vi "7-2.vi"() -> ()   [LabVIEW 2017]
panel:
  out "Gauge":dbl(knob) scale=0.0..10.0
  in  "Stop Button":bool
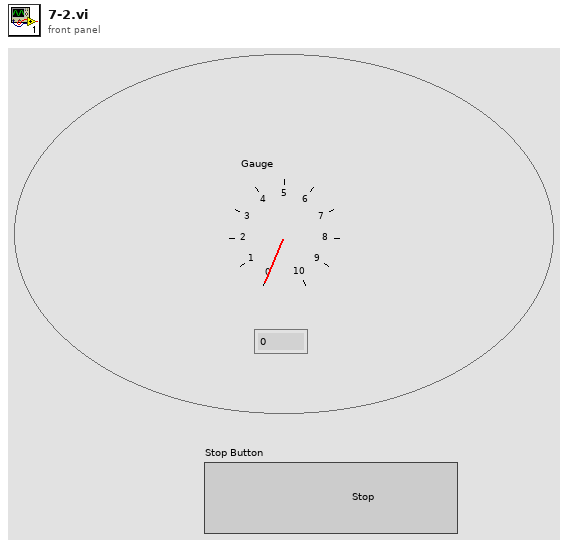
[diagram p1: front panel]
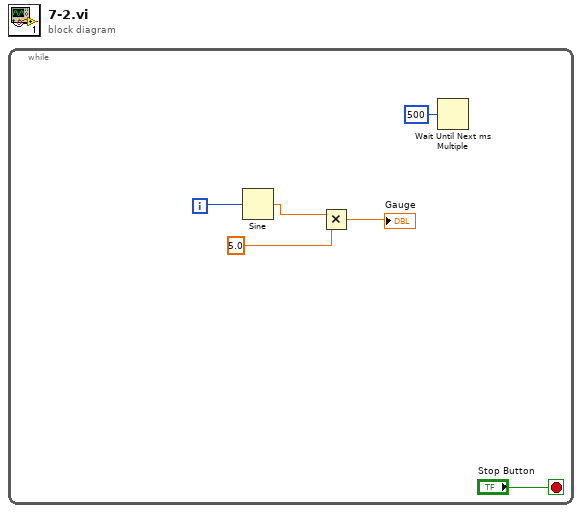
[diagram p0: block diagram]
diagram:
  n1 = while {
    i -> [w5]
    stop <- "Stop Button" stop-if-true
    n2 = Sine(x=w5) -> (sin(x)=w3:dbl)
    n3 = Multiply(x=w3, y=5.0) -> (x*y=→"Gauge":dbl)
    n4 = Wait Until Next ms Multiple(millisecond multiple=u32 500) -> ()  [unwired: 1 out]
  }
